vi "写入表格.vi"(2 "新元素/子数组":string, 8 "错误输入（无错误）":errorcluster, 9 "禁用的索引 (列)":i32, 10 "索引 (行)":i32, 11 "引用":refnum<vi>) -> (0 "错误输出":errorcluster, 3 "引用输出":refnum<vi>)   [LabVIEW 2021]
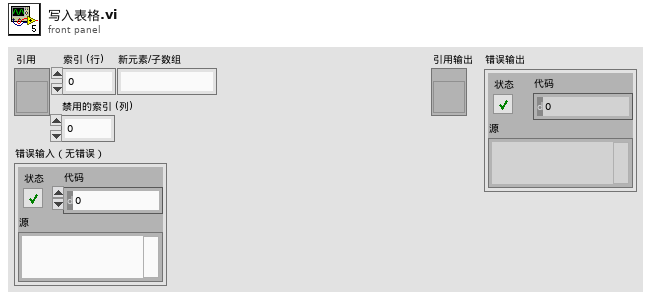
[diagram p1: front panel]
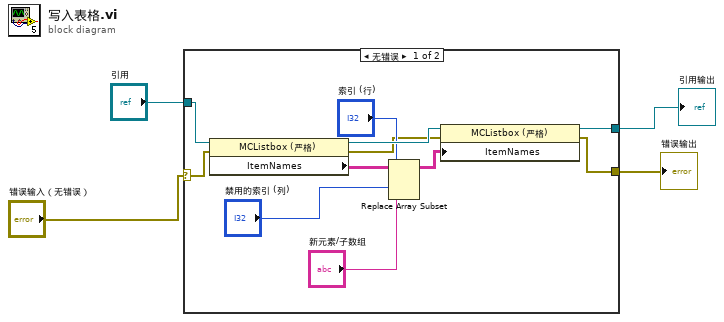
[diagram p0: block diagram]
diagram:
  n1 = case shown="无错误" "错误输入（无错误）" {
    selector: "错误输入（无错误）" -> [w7 w16]
    tunnel: "引用" -> [w15 _]
    tunnel: [w14 _] -> w3
    tunnel: [w6 w16] -> w1
    frame No Error {
      n2 = property class="MCListbox (严格)"(reference=w15, error in=w7) -> (reference out=w12:refnum<vi>, error out=w5:errorcluster, "ItemNames"=w13:string[][])
      n3 = Replace Array Subset(array=w13, new element="新元素/子数组", index (row)="索引 (行)", index (col)="禁用的索引 (列)") -> (w11:string[][])
      n4 = property class="MCListbox (严格)"(reference=w12, error in=w5, "ItemNames"=w11) -> (reference out=w14:refnum<vi>, error out=w6:errorcluster)
    }
    frame Error {
    }
  }
  "引用输出" <- w3
  "错误输出" <- w1
